vi "Encode.vi"(10 "String":string, 11 "Encoding in":refnum<class "Encoding.Base64.lvclass">) -> (2 "Encoded String":string, 3 "Encoding out":refnum<class "Encoding.Base64.lvclass">)   [LabVIEW 2013, in "SMOConfig.lvlib" / "Encoding.Base64.lvclass"]
uses:
  Encoding.Base64.lvclass
  <vilib>/httpClient/LabVIEWHTTPClient.lvlib
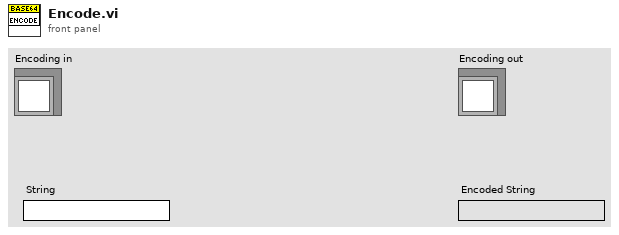
[diagram p1: front panel]
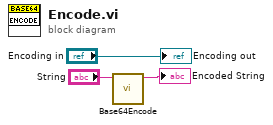
[diagram p0: block diagram]
diagram:
  n1 = call <vilib>:"Base64Encode.vi"("buffer in"="String") -> ("encoded string"=→"Encoded String":string)  [unwired: 9 in, 1 out]
  "Encoding out" <- "Encoding in"
